vi "Read Power Limits (Single).vi"(8 "error in":errorcluster, 9 "Channel Index":i32=1, 11 "Power Limits in":refnum<class "Power Limits.lvclass">) -> (0 "error out":errorcluster, 1 "Lower Power Limit":dbl, 2 "Upper Power Limit":dbl, 3 "Power Limits out":refnum<class "Power Limits.lvclass">, 4 "Changed or First Call?":bool)   [LabVIEW 2023, in "Power Limits.lvclass"]
uses:
  Power Limits.lvclass
  Power Limits.lvclass/Power Limits.ctl
  <vilib>/ADAS Replay HIL/Channels/Tag Wrapper/Polymorphic/Read Channel (Double).vi
  b0de4dd9-b279-4586-9528-e461179a1549.vi
  9f9e3b79-ae2f-4e16-acc3-d25b9e9a90ec.vi
  <vilib>/ADAS Replay HIL/Channels/Tag Wrapper/Polymorphic/Read Channel (Double).vi/b2f764de-0c1e-4784-a155-687fc995a684.vi
  <vilib>/ADAS Replay HIL/Channels/Tag Wrapper/Polymorphic/Read Channel (Double).vi/b2f764de-0c1e-4784-a155-687fc995a684.vi/c28b0ead-42ad-4072-80a2-aca7f2bd7ce3.vi
  <vilib>/ADAS Replay HIL/Channels/Tag Wrapper/Polymorphic/Read Channel (Double).vi/b2f764de-0c1e-4784-a155-687fc995a684.vi/219d0231-d98b-4193-b5cc-84f90e3c9091.vi
  <vilib>/ADAS Replay HIL/Channels/Tag Wrapper/Tag Wrapper.lvlib
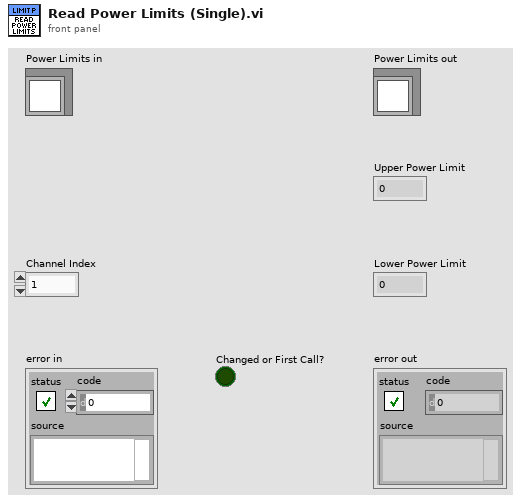
[diagram p1: front panel]
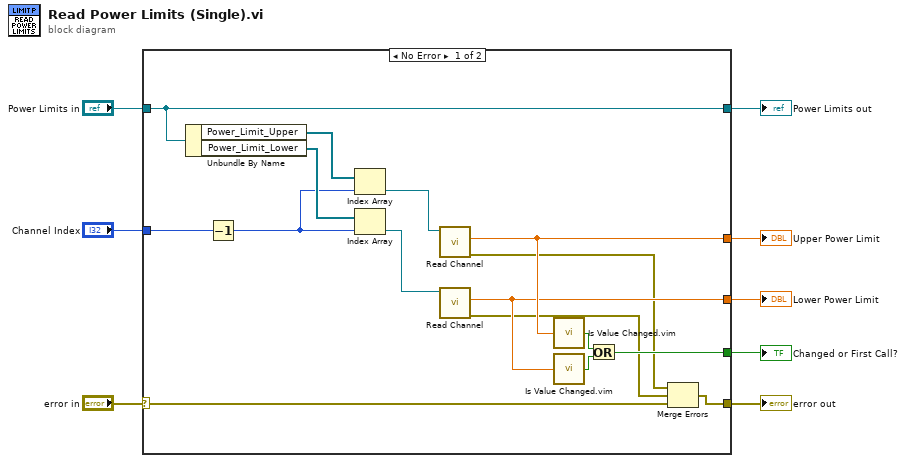
[diagram p0: block diagram]
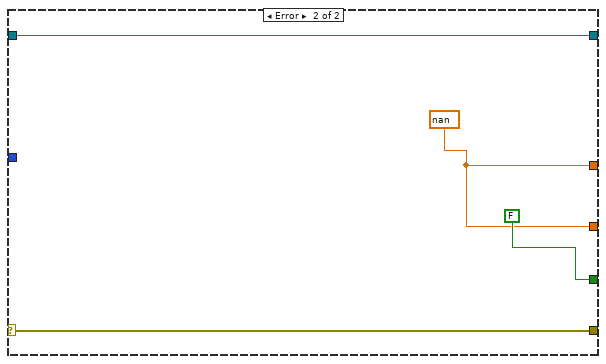
[diagram p2: hidden frame]
diagram:
  n1 = case shown="No Error" "error in" {
    selector: "error in" -> [w18 w28]
    tunnel: [w17 w28] -> w7
    tunnel: [w24 w27] -> w5
    tunnel: "Power Limits in" -> [w24 w27]
    tunnel: [w21 w25] -> w4
    tunnel: [w20 w25] -> w3
    tunnel: [w19 FALSE] -> w2
    tunnel: "Channel Index" -> [w10 _]
    frame No Error {
      n2 = Unbundle By Name(w24) -> ("Power_Limit_Upper"=w22:refnum<k21>[], "Power_Limit_Lower"=w23:refnum<k21>[])
      n3 = Decrement(x=w10) -> (x-1=w9:i32)
      n4 = Index Array(array=w22, index=w9) -> (element=w12:refnum<k21>)
      n5 = Index Array(array=w23, index=w9) -> (element=w11:refnum<k21>)
      n6 = call-poly <vilib>:"Read Channel.vi"("ADAS HIL Channel in"=w12) -> ("error out"=w16:errorcluster, "Value out"=w21:dbl)  [unwired: 7 in, 2 out]
      n7 = call-poly <vilib>:"Read Channel.vi"("ADAS HIL Channel in"=w11) -> ("error out"=w15:errorcluster, "Value out"=w20:dbl)  [unwired: 7 in, 2 out]
      n8 = call "Is Value Changed.vim"("value"=w21) -> ("changed or first call?"=w14:bool)
      n9 = call "Is Value Changed.vim"("value"=w20) -> ("changed or first call?"=w13:bool)
      n10 = Or(x=w14, y=w13) -> (x .or. y?=w19:bool)
      n11 = Merge Errors(w16, w15, w18) -> (w17:errorcluster)
    }
    frame Error {
      w25 = nan ("Value out")
    }
  }
  "error out" <- w7
  "Power Limits out" <- w5
  "Upper Power Limit" <- w4
  "Lower Power Limit" <- w3
  "Changed or First Call?" <- w2
